vi "Sensor Data (Single Reading).vi"(8 "error in (no error)":errorcluster, 9 "Data Source (0:Kelvin)":u16(ring) items=["Kelvin", "Celsius", "Sensor Units"], 10 "Input (0:A)":u16(ring) items=["A", "B", "C", "D"], 11 "VISA resource name":refnum<visa-resource-name>) -> (0 "error out":errorcluster, 2 "Sensor Data":dbl format="%.4f", 3 "VISA resource name out":refnum<visa-resource-name>)   [LabVIEW 2017, in "Lake Shore 336.lvlib"]
doc: "Reads and returns a single sensor reading from the instrument."
uses:
  Lake Shore 336.lvlib
  Instance           1 36Saved   Sensor Data (Single Reading) .vi
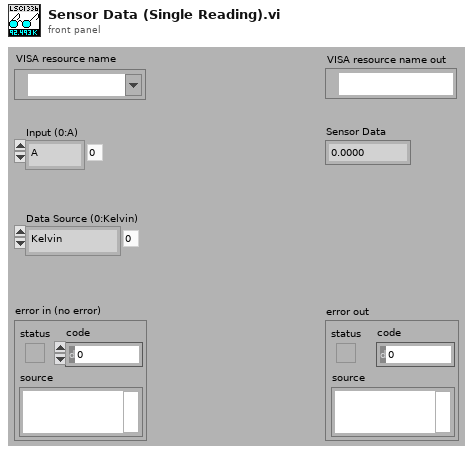
[diagram p1: front panel]
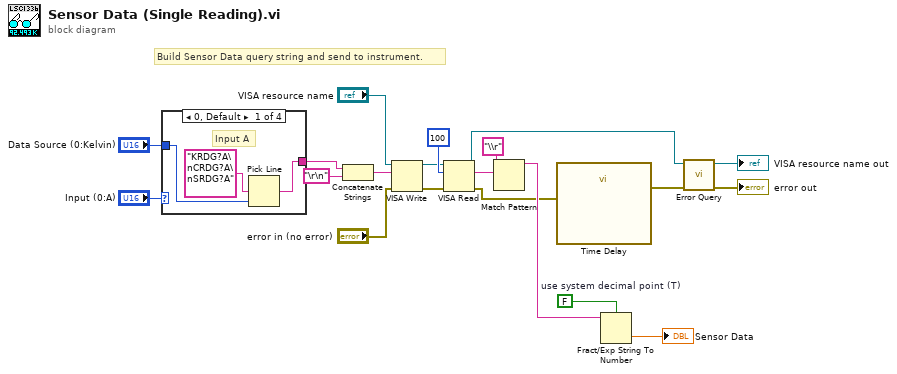
[diagram p0: block diagram]
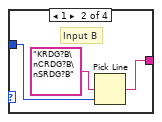
[diagram p2: hidden frame]
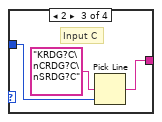
[diagram p3: hidden frame]
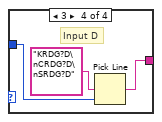
[diagram p4: hidden frame]
diagram:
  w10 = FALSE  # use system decimal point (T)
  # "Build Sensor Data query string and send to instrument."
  n1 = case shown="0, Default" "Input (0:A)" {
    tunnel: "Data Source (0:Kelvin)" -> [w22 w24 w27 w30]
    tunnel: [w21 w25 w28 w31] -> w1
    frame 0, Default {
      # "Input A"
      n2 = Pick Line(multi-line string="KRDG?A\nCRDG?A\nSRDG?A", line index=w22) -> (output string=w21:string)  [unwired: 1 in]
    }
    frame 1 {
      # "Input B"
      n3 = Pick Line(multi-line string="KRDG?B\nCRDG?B\nSRDG?B", line index=w24) -> (output string=w25:string)  [unwired: 1 in]
    }
    frame 2 {
      # "Input C"
      n4 = Pick Line(multi-line string="KRDG?C\nCRDG?C\nSRDG?C", line index=w27) -> (output string=w28:string)  [unwired: 1 in]
    }
    frame 3 {
      # "Input D"
      n5 = Pick Line(multi-line string="KRDG?D\nCRDG?D\nSRDG?D", line index=w30) -> (output string=w31:string)  [unwired: 1 in]
    }
  }
  n6 = Concatenate Strings(w1, "\r\n") -> (w2:string)
  n7 = VISA Write(VISA resource name="VISA resource name", write buffer=w2, error in (no error)="error in (no error)") -> (VISA resource name out=w12:refnum<visa-resource-name>, error out=w11:errorcluster)  [unwired: 1 out]
  n8 = VISA Read(VISA resource name=w12, byte count=100, error in (no error)=w11) -> (VISA resource name out=w16:refnum<visa-resource-name>, read buffer=w14:string, error out=w5:errorcluster)  [unwired: 1 out]
  n9 = Match Pattern(string=w14, regular expression="\\r") -> (before substring=w8:string)  [unwired: 1 in, 3 out]
  n10 = call "Time Delay"("error in (no error)"=w5) -> ("error out"=w6:errorcluster)  [unwired: 10 in]
  n11 = Fract/Exp String To Number(use system decimal point (T)=w10, string=w8) -> (number=→"Sensor Data":dbl)  [unwired: 2 in, 1 out]
  n12 = call "Error Query.vi"("error in (no error)"=w6, "VISA resource name"=w16) -> ("error out"=→"error out":errorcluster, "VISA resource name out"=→"VISA resource name out":refnum<visa-resource-name>)  [unwired: 7 in, 1 out]
